vi "Transport Delay (DBL Array).vi"(2 "initialize":bool, 3 "delay":i32, 5 "Input Points":dbl[](array[numeric]) format="%.2f") -> (1 "Output Points":dbl[](array[numeric]) format="%.2f")   [LabVIEW 2020, in "NI_AdvCtrl_nonlinear.lvlib"]
doc: "LabVIEW no longer supports this VI. You can obtain similar functionality by installing the LabVIEW Simulation Module.\n\nStores input values with an arbitrarily long memory."
uses:
  <vilib>/addons/control/advanced/NI_AdvCtrl_nonlinear.lvlib
  <vilib>/addons/control/advanced/NI_AdvCtrl_continuous linear.lvlib
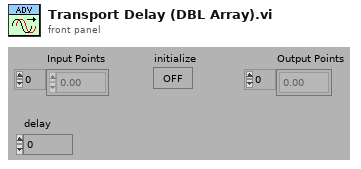
[diagram p1: front panel]
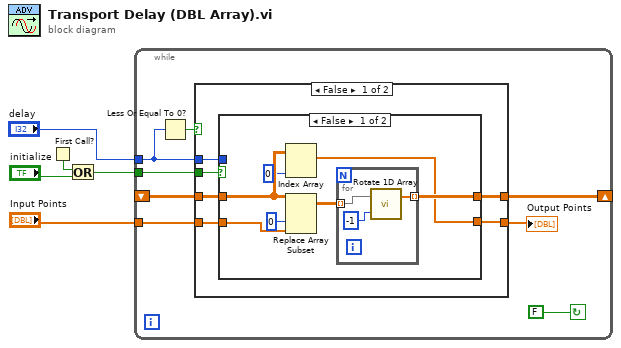
[diagram p0: block diagram]
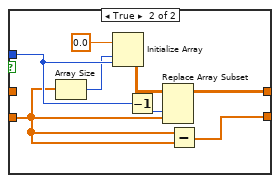
[diagram p2: hidden frame]
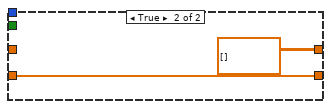
[diagram p3: hidden frame]
diagram:
  n1 = First Call?() -> (First Call?: T/F=w5:bool)
  n2 = Or(x=w5, y="initialize") -> (x .or. y?=w2:bool)
  n3 = while {
    tunnel: "Input Points" -> [w10]
    shift-left: _ -> [w11]
    shift-right: [w12] -> _
    tunnel: "delay" -> [w8]
    tunnel: w2 -> [w13]
    stop <- FALSE continue-if-true
    n4 = Less Or Equal To 0?(x=w8) -> (x <= 0?=w7:bool)
    n5 = case shown="False" w7 {
      tunnel: w13 -> [w19 _]
      tunnel: w8 -> [w18 _]
      tunnel: [w17 dbl[][] []] -> w12
      tunnel: w11 -> [w16 _]
      tunnel: w10 -> [w15 w39]
      tunnel: [w14 w39] -> w6
      frame False {
        n6 = case shown="False" w19 {
          tunnel: w18 -> [_ w34]
          tunnel: [w23 w35] -> w17
          tunnel: w16 -> [w25 _]
          tunnel: w15 -> [w26 w31]
          tunnel: [w22 w30] -> w14
          frame False {
            n7 = Index Array(array=w25, index (col)=0 ("Disabled Index (col)")) -> (element=w22:dbl[])  [unwired: 1 in]
            n8 = Replace Array Subset(array=w25, new element=w26, index (col)=0 ("Disabled Index (col)")) -> (w24:dbl[][])  [unwired: 1 in]
            n9 = for {
              tunnel: w24 -> [w28] mode=indexing
              tunnel: [w29] -> w23 mode=indexing
              n10 = call <vilib>:"Rotate 1D Array.vi"("n"=-1, "array"=w28) -> ("array (last n elements first)"=w29:dbl[])  [unwired: 1 out]
            }
          }
          frame True {
            n11 = Array Size(array=w31) -> (size(s)=w32:i32)
            n12 = Initialize Array(0.0, w32, w34) -> (w36:dbl[][])
            n13 = Decrement(x=w34) -> (x-1=w33:i32)
            n14 = Replace Array Subset(array=w36, new element=w31, index (col)=w33) -> (w35:dbl[][])  [unwired: 1 in]
            n15 = Subtract(x=w31, y=w31) -> (x-y=w30:dbl[])
          }
        }
      }
      frame True {
      }
    }
    "Output Points" <- w6
  }
